vi "cam-box.vi"(8 "error in":errorcluster, 11 "main-national data":T2) -> (0 "error out":errorcluster, 3 "main data out":T2)   [LabVIEW 2019]
uses:
  ctl/main data-national.ctl
  ctl/position set.ctl
panel:
  out "Image Buffer (Image Buffer 5) 2":T1(plugin-control)
  out "Array 2":string[][](array[string])
  out "box array":string[][](array[string])
  out "Image Buffer (Image Buffer 7)":T1(plugin-control)
  out "Image Buffer (Image Buffer 5)":T1(plugin-control)
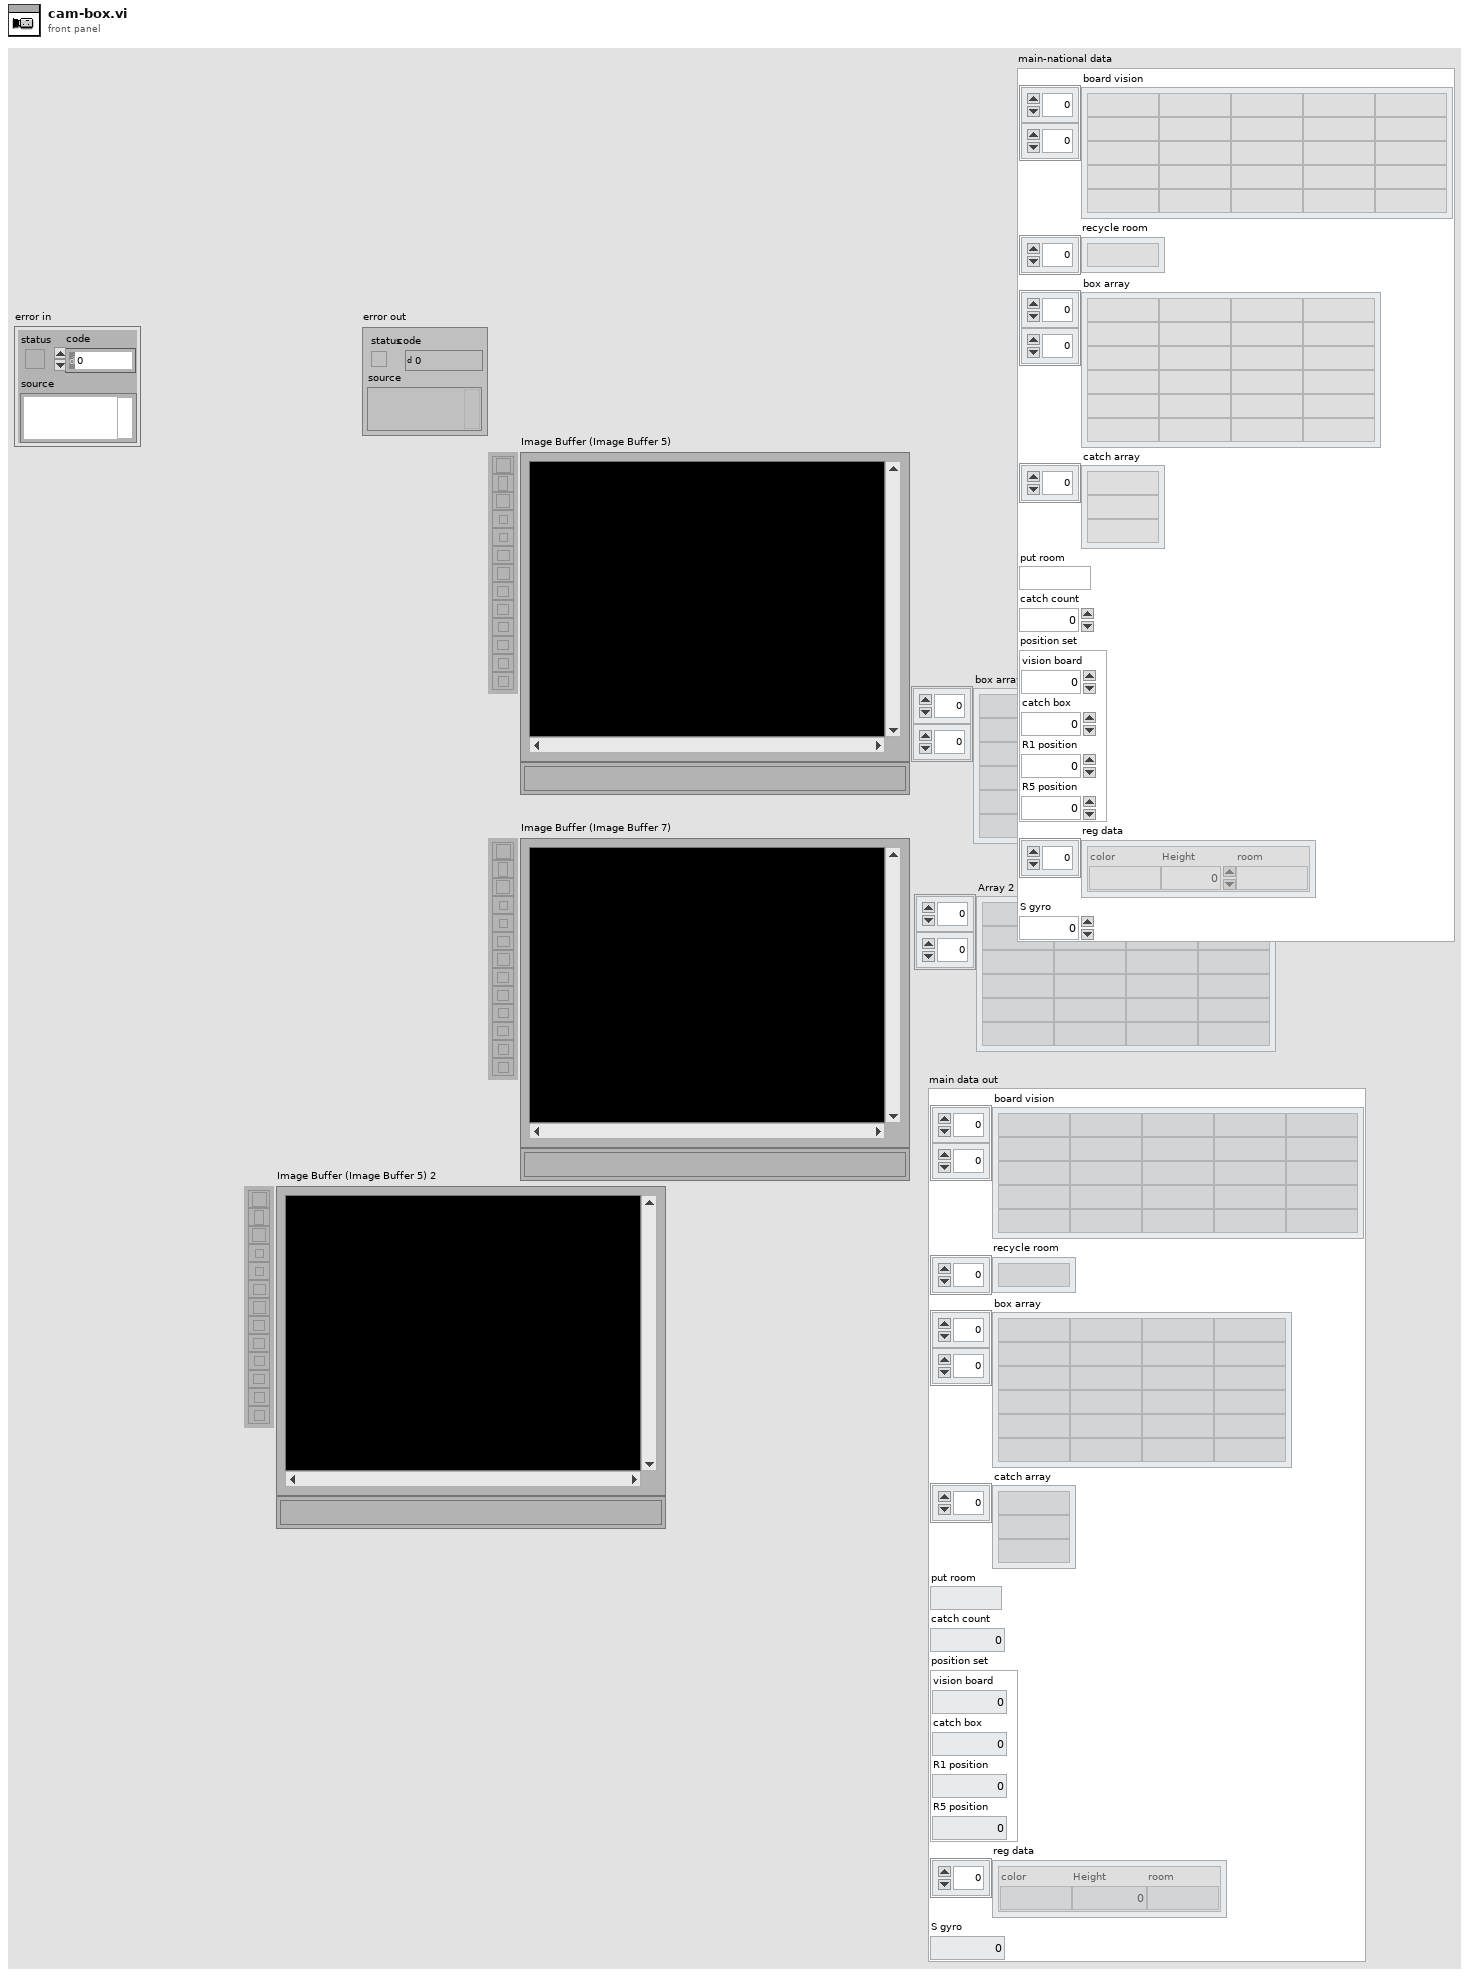
[diagram p1: front panel]
types:
  T1 = typedef "IMAQ Image.ctl" = refnum<image>
  T2 = typedef "main data-national.ctl" = cluster{"board vision":string[][], "recycle room":string[], "box array":string[][], "catch array":string[], "put room":string, "catch count":dbl, "position set":T3, "reg data":cluster{"color":string, "Height":i32, "room":string}[], "S gyro":dbl}
  T3 = typedef "position set.ctl" = cluster{"vision board":dbl, "catch box":dbl, "R1 position":dbl, "R5 position":dbl}
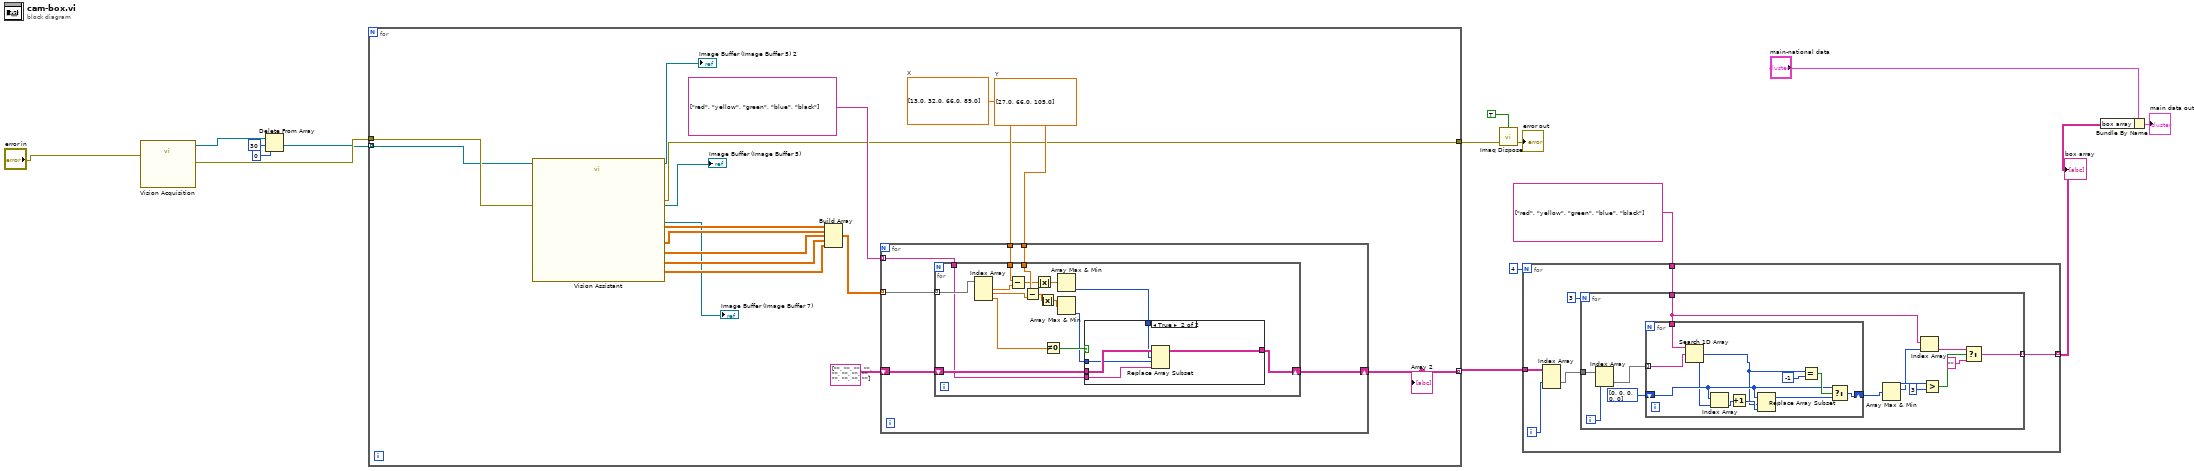
[diagram p0: block diagram]
diagram:
  n1 = call "Vision Acquisition"("error in"="error in") -> ("All Images Out"=w3:T1[], "error out"=w5:errorcluster)  [unwired: 25 in]
  n2 = Delete From Array(array=w3, length=30, index=0) -> (deleted portion=w4:T1[])  [unwired: 1 out]
  n3 = for {
    tunnel: [w21] -> w14 mode=indexing
    tunnel: [w19] -> w11
    tunnel: w5 -> [w18]
    tunnel: w4 -> [w17] mode=indexing
    w28 = dbl[] [27.0, 66.0, 105.0]  # Y
    w29 = dbl[] [13.0, 32.0, 66.0, 89.0]  # X
    n4 = call "Vision Assistant"("Image In"=w17, "error in"=w18) -> ("Image Buffer (Image Buffer 5)"=→"Image Buffer (Image Buffer 5)":T1, "Image Out"=→"Image Buffer (Image Buffer 5) 2":T1, "Particle Measurements (Pixels) (red)"=w22:dbl[][], "Particle Measurements (Pixels) (yellow)"=w23:dbl[][], "Particle Measurements (Pixels) (green)"=w24:dbl[][], "Particle Measurements (Pixels) (blue)"=w25:dbl[][], "Particle Measurements (Pixels) (black)"=w26:dbl[][], "Image Buffer (Image Buffer 21)"=→"Image Buffer (Image Buffer 7)":T1, "error out"=w19:errorcluster)  [unwired: 17 in]
    n5 = Build Array(w22, w23, w24, w25, w26) -> (w30:dbl[][][])
    n6 = for {
      tunnel: string[] ["red", "yellow", "green", "blue", "black"] -> [w37] mode=indexing
      tunnel: w30 -> [w38] mode=indexing
      tunnel: w29 -> [w36]
      tunnel: w28 -> [w35]
      shift-right: [w33] -> w21
      shift-left: string[][] [["", "", ""], ["", "", ""], ["", "", ""], ["", "", ""]] -> [w34]
      n7 = for {
        tunnel: w38 -> [w54] mode=indexing
        tunnel: w37 -> [w40]
        tunnel: w36 -> [w51]
        tunnel: w35 -> [w49]
        shift-right: [w39] -> w33
        shift-left: w34 -> [w43]
        n8 = Index Array(array=w54) -> (element #1=w50:dbl, element #2=w48:dbl, element #3=w52:dbl)  [unwired: 3 in]
        n9 = Subtract(x=w51, y=w50) -> (x-y=w47:dbl[])
        n10 = Subtract(x=w49, y=w48) -> (x-y=w46:dbl[])
        n11 = Absolute Value(x=w47) -> (abs(x)=w44:dbl[])
        n12 = Absolute Value(x=w46) -> (abs(x)=w45:dbl[])
        n13 = Not Equal To 0?(x=w52) -> (x != 0?=w53:bool)
        n14 = Array Max & Min(array=w44) -> (min index (indices)=w42:i32)  [unwired: 3 out]
        n15 = Array Max & Min(array=w45) -> (min index (indices)=w41:i32)  [unwired: 3 out]
        n16 = case shown="True" w53 {
          tunnel: w43 -> [w55 w60]
          tunnel: w42 -> [_ w59]
          tunnel: w41 -> [_ w58]
          tunnel: w40 -> [_ w57]
          tunnel: [w55 w56] -> w39
          frame False {
          }
          frame True {
            n17 = Replace Array Subset(array=w60, new element=w57, index (row)=w59, index (col)=w58) -> (w56:string[][])
          }
        }
      }
    }
    "Array 2" <- w21
  }
  n18 = call "Imaq Dispose"("All Images? (No)"=TRUE, "error in (no error)"=w11) -> ("error out"=→"error out":errorcluster)  [unwired: 4 in]
  n19 = for {
    N: 4 -> [_]
    tunnel: w14 -> [w65]
    tunnel: string[] ["red", "yellow", "green", "blue", "black"] -> [w63]
    tunnel: [w62] -> w8 mode=indexing
    i -> [w61]
    n20 = Index Array(array=w65, index (dim 1)=w61) -> (element=w64:string[][])  [unwired: 2 in]
    n21 = for {
      N: 3 -> [_]
      tunnel: w64 -> [w79]
      tunnel: w63 -> [w72]
      tunnel: [w69] -> w62 mode=indexing
      i -> [w67]
      n22 = Index Array(array=w79, index (col)=w67) -> (element=w78:string[])  [unwired: 1 in]
      n23 = for {
        tunnel: w78 -> [w88] mode=indexing
        tunnel: w72 -> [w89]
        shift-right: [w80] -> w76
        shift-left: i32[] [0, 0, 0, 0, 0] -> [w84]
        n24 = Search 1D Array(1D array=w89, element=w88) -> (index of element=w82:i32)  [unwired: 1 in]
        n25 = Index Array(array=w84, index=w82) -> (element=w85:i32)
        n26 = Increment(x=w85) -> (x+1=w83:i32)
        n27 = Replace Array Subset(array=w84, new element=w83, index=w82) -> (w81:i32[])
        n28 = Equal?(x=w82, y=-1) -> (x = y?=w86:bool)
        n29 = Select(t=w84, s=w86, f=w81) -> (s? t:f=w80:i32[])
      }
      n30 = Array Max & Min(array=w76) -> (max value=w71:i32, max index (indices)=w68:i32)  [unwired: 2 out]
      n31 = Index Array(array=w72, index=w68) -> (element=w70:string)
      n32 = Greater?(x=w71, y=3) -> (0:w74:bool)
      n33 = Select(t=w70, s=w74, f="") -> (s? t:f=w69:string)
    }
  }
  "box array" <- w8
  n34 = Bundle By Name(cluster="main-national data", "box array"=w8) -> (→"main data out":T2)
